vi "WSVCAP SHL FPGA LL I2C Write CLK.vi"(0 "Bit In":bool, 11 "error in (no error)":errorcluster, 12 "UUT Set (0/1 (Legacy)":u8, 14 "Socket Mask":u64 format="%08x") -> (15 "error out":errorcluster)   [LabVIEW 2017]
uses:
  WSVCAP SHL FPGA LL I2C Debug Global.vi
  <vilib>/eio/EIONode/EIONode.xnode
  <vilib>/rvi/eio/common/nirviEmuTemplateMethod_errors.vi
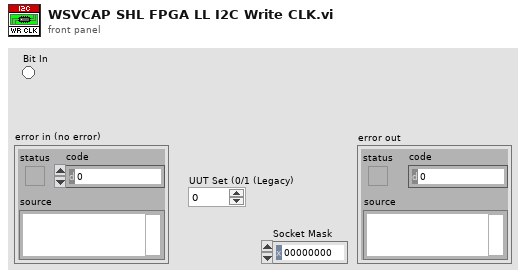
[diagram p1: front panel]
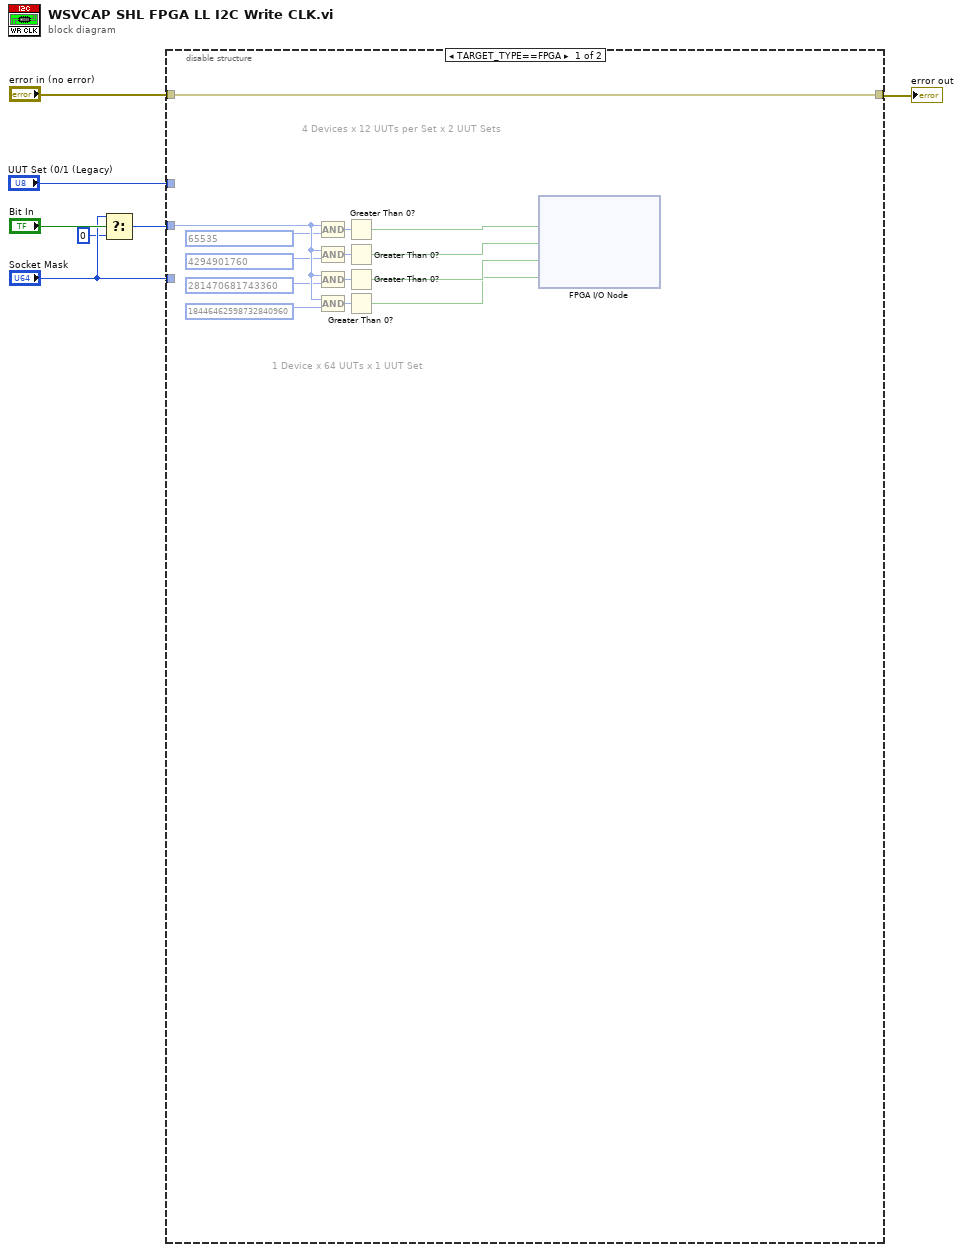
[diagram p0: block diagram]
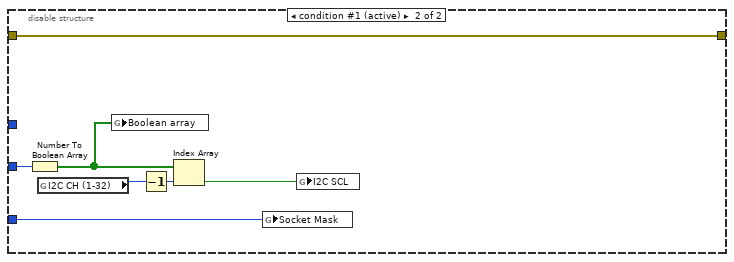
[diagram p2: hidden frame]
diagram:
  n1 = Select(t="Socket Mask", s="Bit In", f=u64 0) -> (s? t:f=w1:u64)
  n2 = disable-structure shown="TARGET_TYPE==FPGA" {
    disable-tunnel: w1 -> [w21 w24]
    disable-tunnel: [w20 w28] -> w7
    disable-tunnel: "error in (no error)" -> [w20 w28]
    disable-tunnel: "Socket Mask" -> [_ w22]
    disable-tunnel: "UUT Set (0/1 (Legacy)" -> [_ _]
    frame condition #0 {
      # "1 Device x 64 UUTs x 1 UUT Set"
      # "4 Devices x 12 UUTs per Set x 2 UUT Sets"
      n3 = Compound Arithmetic op=AND(w21, u64 65535) -> (w19:u64)
      n4 = Compound Arithmetic op=AND(w21, u64 4294901760) -> (w18:u64)
      n5 = Compound Arithmetic op=AND(w21, u64 281470681743360) -> (w17:u64)
      n6 = Compound Arithmetic op=AND(w21, u64 18446462598732840960) -> (w16:u64)
      n7 = Greater Than 0?(x=w19) -> (x > 0?=w15:bool)
      n8 = Greater Than 0?(x=w18) -> (x > 0?=w14:bool)
      n9 = Greater Than 0?(x=w17) -> (x > 0?=w13:bool)
      n10 = Greater Than 0?(x=w16) -> (x > 0?=w12:bool)
      n11 = xnode "FPGA I/O Node"("I2C_SCL_S1-S16"=w15, "I2C_SCL_S17-32"=w14, "I2C_SCL_S33-48"=w13, "I2C_SCL_S49-64"=w12) -> ()  [unwired: 5 in, 5 out]
    }
    frame condition #1 (active) {
      n12 = Number To Boolean Array(number=w24) -> (Boolean array=w23:bool[])
      n13 = global read "WSVCAP SHL FPGA LL I2C Debug Global.vi" "I2C CH (1-32)"() -> (w26:i32)
      n14 = global write "WSVCAP SHL FPGA LL I2C Debug Global.vi" "Boolean array"(w23) -> ()
      n15 = Decrement(x=w26) -> (x-1=w25:i32)
      n16 = Index Array(array=w23, index=w25) -> (element=w27:bool)
      n17 = global write "WSVCAP SHL FPGA LL I2C Debug Global.vi" "Socket Mask"(w22) -> ()
      n18 = global write "WSVCAP SHL FPGA LL I2C Debug Global.vi" "I2C SCL"(w27) -> ()
    }
  }
  "error out" <- w7
